vi "Get_Complete.vi"(0 ".NET Refnum in":refnum<k24>, 5 "error in (no error)":errorcluster) -> (14 ".NET Refnum out":refnum<k24>, 19 "error out":errorcluster)   [LabVIEW 2016]
uses:
  System.Windows.Forms
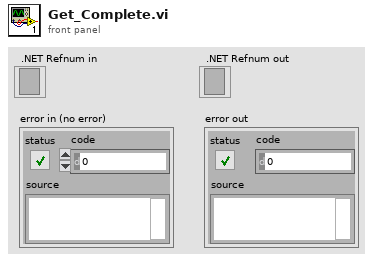
[diagram p1: front panel]
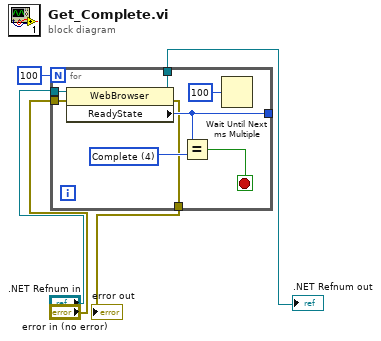
[diagram p0: block diagram]
diagram:
  n1 = for {
    N: 100 -> [_]
    tunnel: ".NET Refnum in" -> [w13]
    tunnel: [w12] -> _
    tunnel: [w8] -> w5
    tunnel: "error in (no error)" -> [w7]
    tunnel: [w6] -> w4
    stop <- w10 stop-if-true
    w11 = 4 items=["Uninitialized", "Loading", "Loaded", "Interactive", "Complete"] ("ReadyState")
    n2 = property class="WebBrowser"(reference=w13, error in=w7) -> (reference out=w8:refnum<k24>, error out=w6:errorcluster, "ReadyState"=w12:i32)
    n3 = Equal?(x=w12, y=w11) -> (x = y?=w10:bool)
    n4 = Wait Until Next ms Multiple(millisecond multiple=u32 100) -> ()  [unwired: 1 out]
  }
  ".NET Refnum out" <- w5
  "error out" <- w4
